vi "_readLabel_fromLabelList_wmg.vi"(0 "input_str_SN":string="8SSC10G59338L1DG5AN0004", 1 "input_str_PN":string="L01HE006-SD-R") -> (2 "show_str_SN":string, 3 "show_int_SN":i32, 4 "show_string_yydddXXXX":string, 5 "show_date":timestamp format="%<%X\n%x>T")   [LabVIEW 2011]
panel:
  in  "midVar_date_2":timestamp
  in  "midVar_date_1":timestamp
  # "周日是一周的第0天"
  # "1904050897/Z00A2R1543S500016\n0       5       10         17     22\nL99SF014-SD-H"
  # "8SSC10G59338L1DG5AN0004\nL01HE006-SD-R"
  # "1904050897/Z00A2R1543S500016\n0       5       10         17     22\nL99SF014-SD-H\n\n1543S5经本程序计算得到2015/10/23 296"
  # "8SSC10G59338L1DG5AN0004\n\nL01HE006-SD-R\n5AN经本程序计算得到2015/10/22 295\n\n8SSC10G59338L1DG5110004\nL01HE006-SD-R\n5AN经本程序计算得到2015/1/1 1"
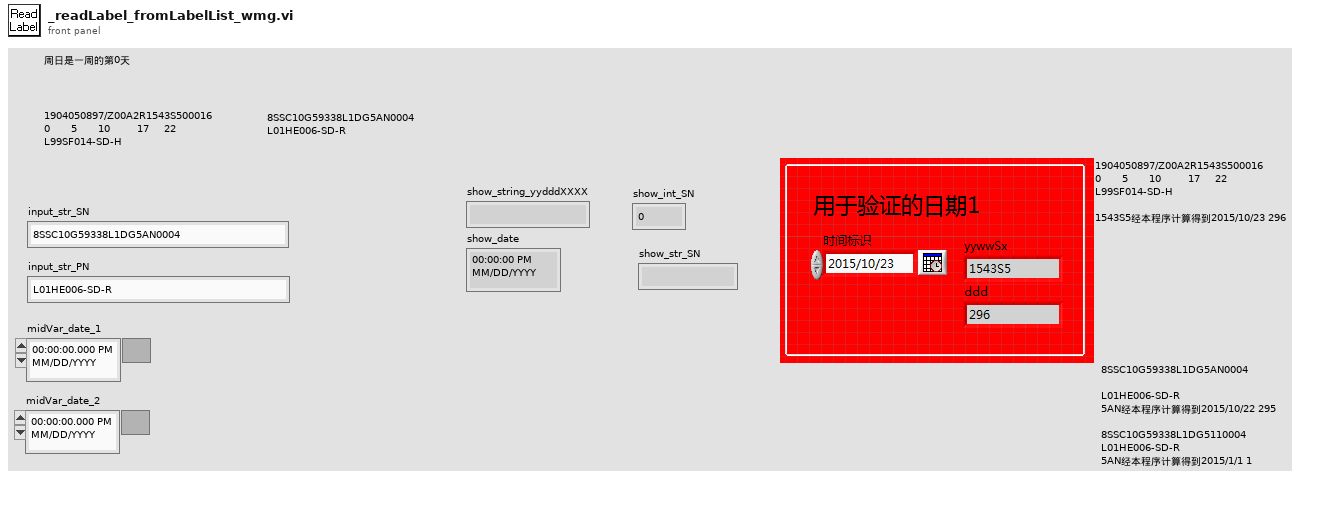
[diagram p1: front panel]
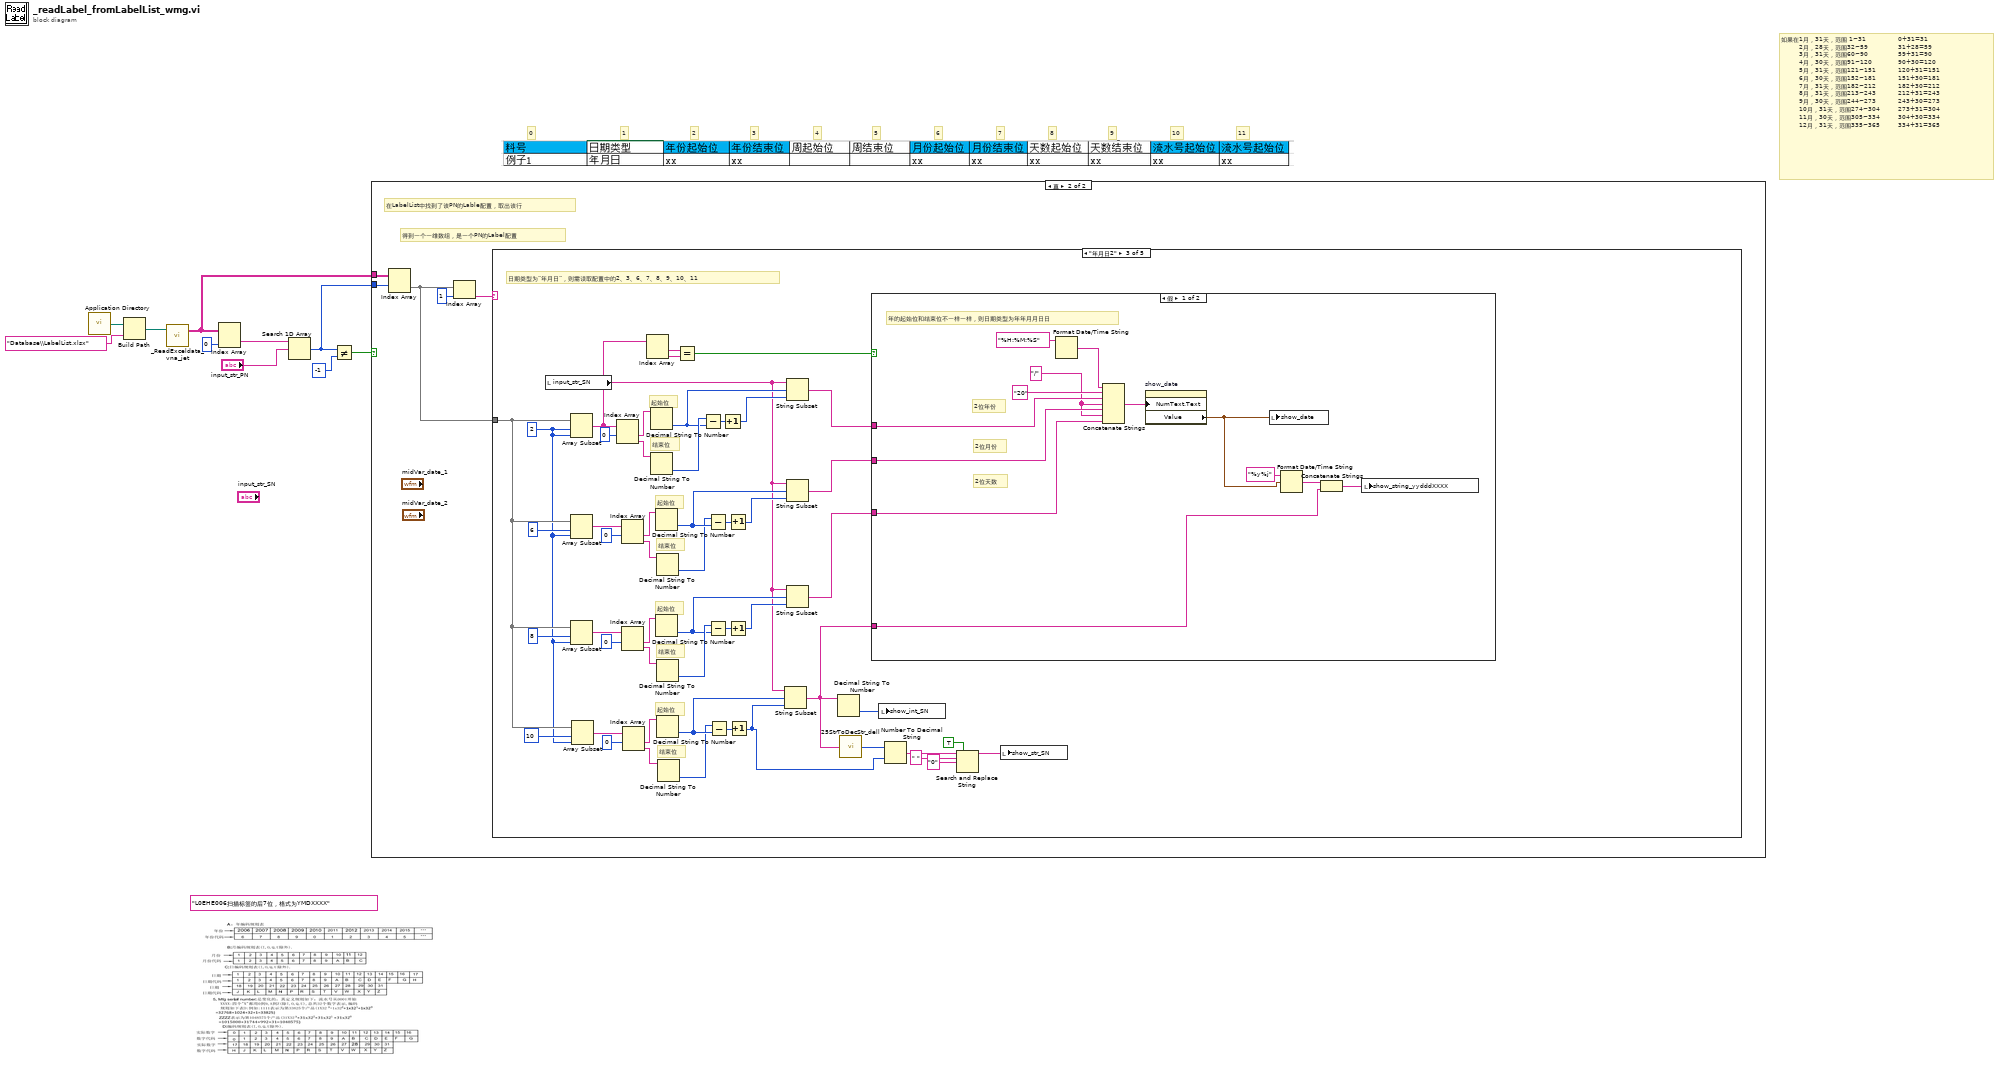
[diagram p0: block diagram]
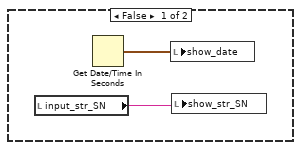
[diagram p2: hidden frame]
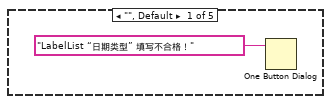
[diagram p3: hidden frame]
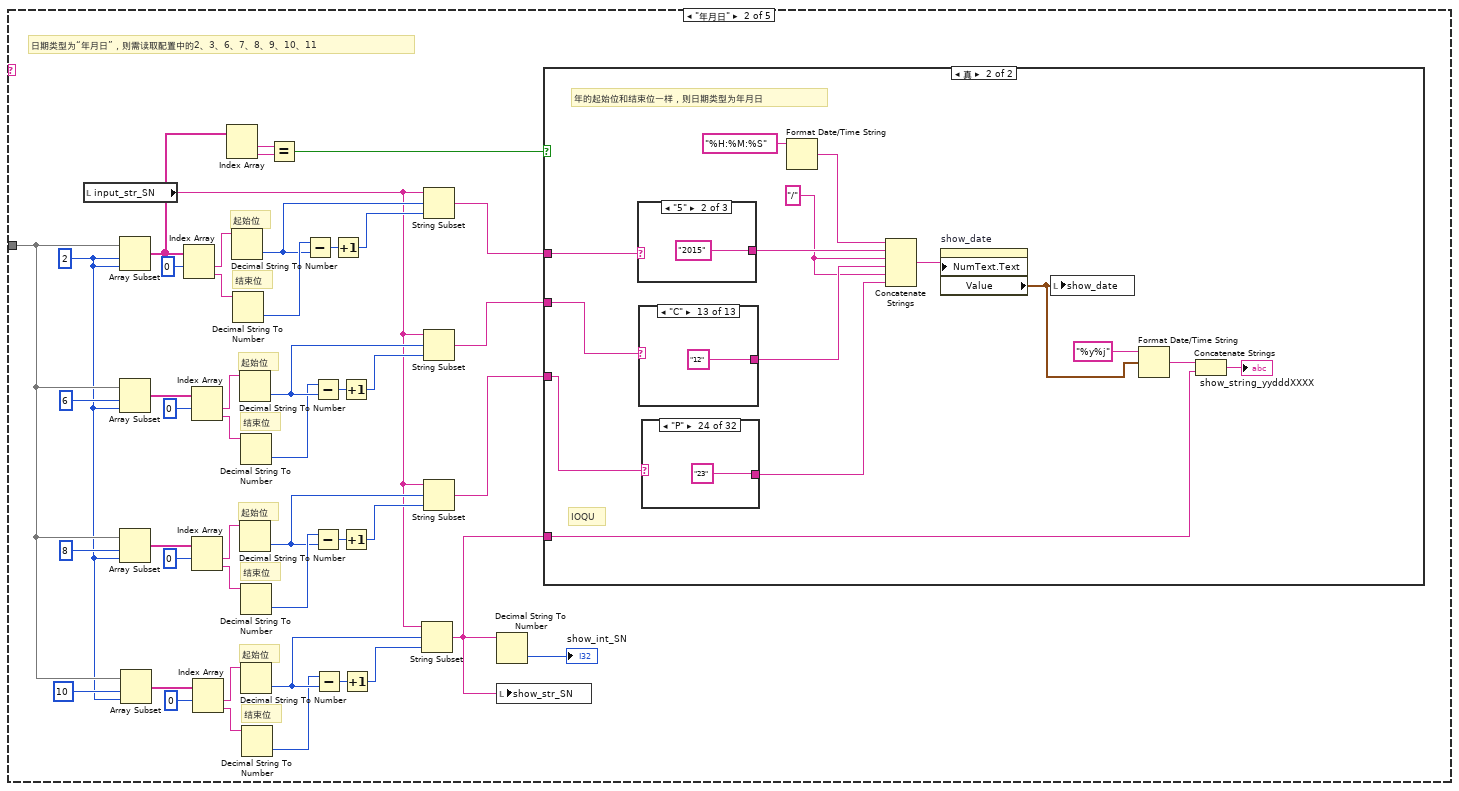
[diagram p4: hidden frame]
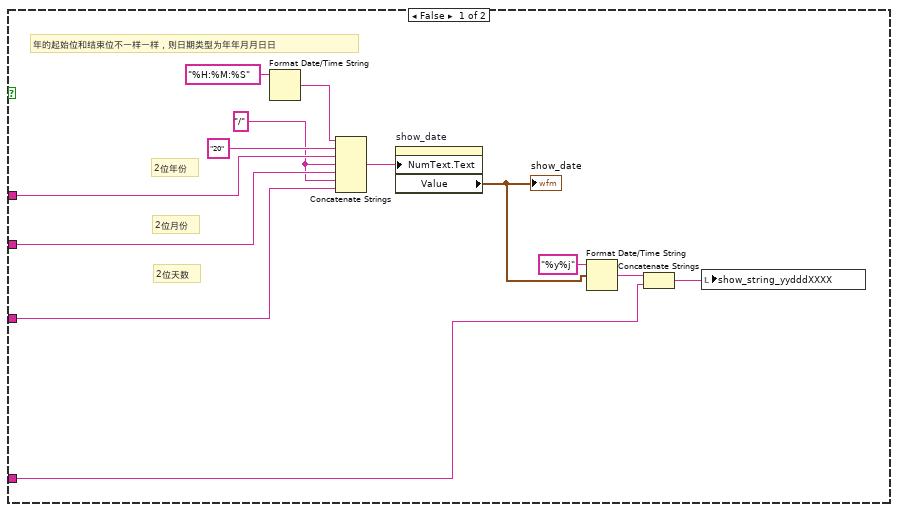
[diagram p5: hidden frame]
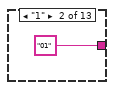
[diagram p7: hidden frame]
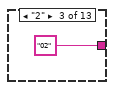
[diagram p8: hidden frame]
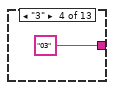
[diagram p9: hidden frame]
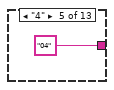
[diagram p10: hidden frame]
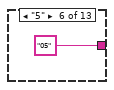
[diagram p11: hidden frame]
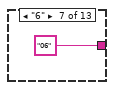
[diagram p12: hidden frame]
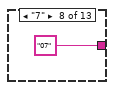
[diagram p13: hidden frame]
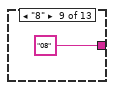
[diagram p14: hidden frame]
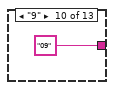
[diagram p15: hidden frame]
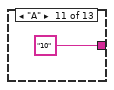
[diagram p16: hidden frame]
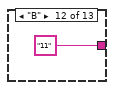
[diagram p17: hidden frame]
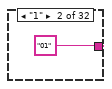
[diagram p19: hidden frame]
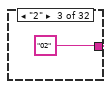
[diagram p20: hidden frame]
diagram:
  (unwired) "L0EHE006扫描标签的后7位，格式为YMDXXXX"
  # "如果在1月，31天，范围 1~31                0+31=31\n         2月，28天，范围32~59               31+28=59\n         3月，31天，范围60~90               59+31=90\n         4月，30天，范围91~120             90+30=120\n         5月，31天，范围121~151           120+31=151\n         6月，30天，范围152~181           151+30=181\n         7月，31天，范围182~212           182+30=212\n         8月，31天，范围213~243           212+31=243\n         9月，30天，范围244~273           243+30=273\n         10月，31天，范围274~304         273+31=304\n         11月，30天，范围305~334         304+30=334\n         12月，31天，范围335~365         334+31=365"
  # "11"
  # "10"
  # "9"
  # "8"
  # "7"
  # "6"
  # "5"
  # "4"
  # "3"
  # "2"
  # "1"
  # "0"
  n1 = call <vilib>:"Application Directory.vi"() -> ("Application Directory"=w10:path)
  n2 = Build Path(base path=w10, name or relative path="Database\\LabelList.xlsx") -> (appended path=w8:path)
  n3 = call "_ReadExceldata_vna_jet.vi"("路径"=w8) -> ("数据"=w2:string[][])  [unwired: 4 in]
  n4 = Index Array(array=w2, index (col)=0 ("禁用的索引 (列)")) -> (element=w6:string[])  [unwired: 1 in]
  n5 = Search 1D Array(1D array=w6, element="input_str_PN") -> (index of element=w1:i32)  [unwired: 1 in]
  n6 = Not Equal?(x=w1, y=-1) -> (x != y?=w3:bool)
  n7 = case shown="真" w3 {
    tunnel: w2 -> [_ w17]
    tunnel: w1 -> [_ w16]
    frame False {
      n8 = local read "input_str_SN"() -> (w11:string)
      n9 = Get Date/Time In Seconds() -> (seconds since 1Jan1904=w12:timestamp)
      n10 = local write "show_date"(w12) -> ()
      n11 = local write "show_str_SN"(w11) -> ()
    }
    frame True {
      # "得到一个一维数组，是一个PN的Label配置"
      # "在LabelList中找到了该PN的Lable配置，取出该行"
      n12 = Index Array(array=w17, index (row)=w16) -> (element=w13:string[])  [unwired: 1 in]
      n13 = Index Array(array=w13, index=1 ("索引")) -> (element=w14:string)
      n14 = case shown="\"年月日2\"" w14 {
        tunnel: w13 -> [_ w61 w186 w333 w357]
        frame "", Default {
          n15 = One Button Dialog(message="LabelList “日期类型” 填写不合格！") -> ()  [unwired: 1 in, 1 out]
        }
        frame "年月日" {
          w60 = 2 ("索引")
          # "结束位"
          # "起始位"
          # "结束位"
          # "起始位"
          # "结束位"
          # "起始位"
          # "结束位"
          # "起始位"
          # "日期类型为“年月日”，则需读取配置中的2、3、6、7、8、9、10、11"
          n16 = local read "input_str_SN"() -> (w21:string)
          n17 = Array Subset(array=w61, index=w60, length=w60) -> (w55:string[])
          n18 = Array Subset(array=w61, index=6 ("索引"), length=w60) -> (w42:string[])
          n19 = Array Subset(array=w61, index=8 ("索引"), length=w60) -> (w34:string[])
          n20 = Array Subset(array=w61, index=10 ("索引"), length=w60) -> (w22:string[])
          n21 = Index Array(array=w55, index #1=0 ("索引")) -> (element #1=w54:string, element #2=w53:string)  [unwired: 1 in]
          n22 = Index Array(array=w42, index #1=0 ("索引")) -> (element #1=w44:string, element #2=w45:string)  [unwired: 1 in]
          n23 = Index Array(array=w34, index #1=0 ("索引")) -> (element #1=w35:string, element #2=w39:string)  [unwired: 1 in]
          n24 = Index Array(array=w22, index #1=0 ("索引")) -> (element #1=w28:string, element #2=w24:string)  [unwired: 1 in]
          n25 = Index Array(array=w55) -> (element #1=w59:string, element #2=w58:string)  [unwired: 2 in]
          n26 = Decimal String To Number(string=w54) -> (number=w51:i32)  [unwired: 2 in, 1 out]
          n27 = Decimal String To Number(string=w53) -> (number=w52:i32)  [unwired: 2 in, 1 out]
          n28 = Decimal String To Number(string=w44) -> (number=w47:i32)  [unwired: 2 in, 1 out]
          n29 = Decimal String To Number(string=w35) -> (number=w37:i32)  [unwired: 2 in, 1 out]
          n30 = Decimal String To Number(string=w45) -> (number=w46:i32)  [unwired: 2 in, 1 out]
          n31 = Decimal String To Number(string=w39) -> (number=w38:i32)  [unwired: 2 in, 1 out]
          n32 = Decimal String To Number(string=w28) -> (number=w26:i32)  [unwired: 2 in, 1 out]
          n33 = Decimal String To Number(string=w24) -> (number=w25:i32)  [unwired: 2 in, 1 out]
          n34 = Equal?(x=w59, y=w58) -> (x = y?=w57:bool)
          n35 = Subtract(x=w52, y=w51) -> (x-y=w56:i32)
          n36 = Subtract(x=w46, y=w47) -> (x-y=w43:i32)
          n37 = Subtract(x=w38, y=w37) -> (x-y=w40:i32)
          n38 = Subtract(x=w25, y=w26) -> (x-y=w23:i32)
          n39 = Increment(x=w56) -> (x+1=w50:i32)
          n40 = Increment(x=w43) -> (x+1=w48:i32)
          n41 = Increment(x=w40) -> (x+1=w36:i32)
          n42 = Increment(x=w23) -> (x+1=w27:i32)
          n43 = String Subset(string=w21, offset (0)=w26, length (rest)=w27) -> (substring=w19:string)
          n44 = String Subset(string=w21, offset (0)=w51, length (rest)=w50) -> (substring=w49:string)
          n45 = String Subset(string=w21, offset (0)=w47, length (rest)=w48) -> (substring=w41:string)
          n46 = String Subset(string=w21, offset (0)=w37, length (rest)=w36) -> (substring=w30:string)
          n47 = Decimal String To Number(string=w19) -> (number=→"show_int_SN":i32)  [unwired: 2 in, 1 out]
          n48 = local write "show_str_SN"(w19) -> ()
          n49 = case shown="真" w57 {
            tunnel: w49 -> [w76 w92]
            tunnel: w41 -> [w75 w90]
            tunnel: w30 -> [w73 w91]
            tunnel: w19 -> [w65 w78]
            frame False {
              w74 = "/"
              # "年的起始位和结束位不一样一样，则日期类型为年年月月日日"
              # "2位天数"
              # "2位月份"
              # "2位年份"
              n50 = Format Date/Time String(time format string (%c)="%H:%M:%S" ("时间格式字符串(%c)")) -> (date/time string=w71:string)  [unwired: 2 in]
              n51 = Concatenate Strings(w71, "20", w76, w74, w75, w74, w73) -> (w70:string)
              n52 = property on="show_date" class="AbsTime (严格)"("NumText.Text"=w70) -> ("Value"=w66:timestamp)  [unwired: 2 in, 2 out]
              "show_date" <- w66
              n53 = Format Date/Time String(time format string (%c)="%y%j" ("时间格式字符串(%c)"), seconds (now)=w66) -> (date/time string=w68:string)  [unwired: 1 in]
              n54 = Concatenate Strings(w68, w65) -> (w69:string)
              n55 = local write "show_string_yydddXXXX"(w69) -> ()
            }
            frame True {
              w85 = "/"
              # "IOQU"
              # "年的起始位和结束位一样，则日期类型为年月日"
              n56 = case shown="\"5\"" w92 {
                tunnel: [_ "2015" "2016"] -> w89
                frame Default {
                }
                frame "5" {
                }
                frame "6" {
                }
              }
              n57 = case shown="\"C\"" w90 {
                tunnel: [_ "01" "02" "03" "04" "05" "06" "07" "08" "09" "10" "11" "12"] -> w86
                frame "", Default {
                }
                frame "1" {
                }
                frame "2" {
                }
                frame "3" {
                }
                frame "4" {
                }
                frame "5" {
                }
                frame "6" {
                }
                frame "7" {
                }
                frame "8" {
                }
                frame "9" {
                }
                frame "A" {
                }
                frame "B" {
                }
                frame "C" {
                }
              }
              n58 = case shown="\"P\"" w91 {
                tunnel: [_ "01" "02" "03" "04" "05" "06" "07" "08" "09" "10" "11" "12" "13" "14" "15" "16" "17" "18" "19" "20" "21" "22" "23" "24" "25" "26" "27" "28" "29" "30" "31"] -> w84
                frame "", Default {
                }
                frame "1" {
                }
                frame "2" {
                }
                frame "3" {
                }
                frame "4" {
                }
                frame "5" {
                }
                frame "6" {
                }
                frame "7" {
                }
                frame "8" {
                }
                frame "9" {
                }
                frame "A" {
                }
                frame "B" {
                }
                frame "C" {
                }
                frame "D" {
                }
                frame "E" {
                }
                frame "F" {
                }
                frame "G" {
                }
                frame "H" {
                }
                frame "J" {
                }
                frame "K" {
                }
                frame "L" {
                }
                frame "M" {
                }
                frame "N" {
                }
                frame "P" {
                }
                frame "R" {
                }
                frame "S" {
                }
                frame "T" {
                }
                frame "V" {
                }
                frame "W" {
                }
                frame "X" {
                }
                frame "Y" {
                }
                frame "Z" {
                }
              }
              n59 = Format Date/Time String(time format string (%c)="%H:%M:%S" ("时间格式字符串(%c)")) -> (date/time string=w87:string)  [unwired: 2 in]
              n60 = Concatenate Strings(w87, w89, w85, w86, w85, w84) -> (w83:string)
              n61 = property on="show_date" class="AbsTime (严格)"("NumText.Text"=w83) -> ("Value"=w79:timestamp)  [unwired: 2 in, 2 out]
              n62 = local write "show_date"(w79) -> ()
              n63 = Format Date/Time String(time format string (%c)="%y%j" ("时间格式字符串(%c)"), seconds (now)=w79) -> (date/time string=w81:string)  [unwired: 1 in]
              n64 = Concatenate Strings(w81, w78) -> (→"show_string_yydddXXXX":string)
            }
          }
        }
        frame "年月日2" {
          w185 = 2 ("索引")
          # "结束位"
          # "起始位"
          # "结束位"
          # "起始位"
          # "结束位"
          # "起始位"
          # "结束位"
          # "起始位"
          # "日期类型为“年月日”，则需读取配置中的2、3、6、7、8、9、10、11"
          n65 = local read "input_str_SN"() -> (w147:string)
          n66 = Array Subset(array=w186, index=w185, length=w185) -> (w180:string[])
          n67 = Array Subset(array=w186, index=6 ("索引"), length=w185) -> (w167:string[])
          n68 = Array Subset(array=w186, index=8 ("索引"), length=w185) -> (w159:string[])
          n69 = Array Subset(array=w186, index=10 ("索引"), length=w185) -> (w148:string[])
          n70 = Index Array(array=w180, index #1=0 ("索引")) -> (element #1=w179:string, element #2=w178:string)  [unwired: 1 in]
          n71 = Index Array(array=w167, index #1=0 ("索引")) -> (element #1=w169:string, element #2=w170:string)  [unwired: 1 in]
          n72 = Index Array(array=w159, index #1=0 ("索引")) -> (element #1=w160:string, element #2=w164:string)  [unwired: 1 in]
          n73 = Index Array(array=w148, index #1=0 ("索引")) -> (element #1=w153:string, element #2=w150:string)  [unwired: 1 in]
          n74 = Index Array(array=w180) -> (element #1=w184:string, element #2=w183:string)  [unwired: 2 in]
          n75 = Decimal String To Number(string=w179) -> (number=w176:i32)  [unwired: 2 in, 1 out]
          n76 = Decimal String To Number(string=w178) -> (number=w177:i32)  [unwired: 2 in, 1 out]
          n77 = Decimal String To Number(string=w169) -> (number=w172:i32)  [unwired: 2 in, 1 out]
          n78 = Decimal String To Number(string=w160) -> (number=w162:i32)  [unwired: 2 in, 1 out]
          n79 = Decimal String To Number(string=w170) -> (number=w171:i32)  [unwired: 2 in, 1 out]
          n80 = Decimal String To Number(string=w164) -> (number=w163:i32)  [unwired: 2 in, 1 out]
          n81 = Decimal String To Number(string=w153) -> (number=w152:i32)  [unwired: 2 in, 1 out]
          n82 = Decimal String To Number(string=w150) -> (number=w151:i32)  [unwired: 2 in, 1 out]
          n83 = Equal?(x=w184, y=w183) -> (x = y?=w182:bool)
          n84 = Subtract(x=w177, y=w176) -> (x-y=w181:i32)
          n85 = Subtract(x=w171, y=w172) -> (x-y=w168:i32)
          n86 = Subtract(x=w163, y=w162) -> (x-y=w165:i32)
          n87 = Subtract(x=w151, y=w152) -> (x-y=w149:i32)
          n88 = Increment(x=w181) -> (x+1=w175:i32)
          n89 = Increment(x=w168) -> (x+1=w173:i32)
          n90 = Increment(x=w165) -> (x+1=w161:i32)
          n91 = Increment(x=w149) -> (x+1=w143:i32)
          n92 = String Subset(string=w147, offset (0)=w152, length (rest)=w143) -> (substring=w146:string)
          n93 = String Subset(string=w147, offset (0)=w176, length (rest)=w175) -> (substring=w174:string)
          n94 = String Subset(string=w147, offset (0)=w172, length (rest)=w173) -> (substring=w166:string)
          n95 = String Subset(string=w147, offset (0)=w162, length (rest)=w161) -> (substring=w155:string)
          n96 = Decimal String To Number(string=w146) -> (number=w145:i32)  [unwired: 2 in, 1 out]
          n97 = call "25StrToDecStr_dell.vi"("input_str_hex"=w146) -> ("数值"=w144:i32)
          n98 = case shown="假" w182 {
            tunnel: w174 -> [w201 w217]
            tunnel: w166 -> [w200 w215]
            tunnel: w155 -> [w198 w216]
            tunnel: w146 -> [w192 w204]
            frame False {
              w199 = "/"
              # "年的起始位和结束位不一样一样，则日期类型为年年月月日日"
              # "2位天数"
              # "2位月份"
              # "2位年份"
              n99 = Format Date/Time String(time format string (%c)="%H:%M:%S" ("时间格式字符串(%c)")) -> (date/time string=w196:string)  [unwired: 2 in]
              n100 = Concatenate Strings(w196, "20", w201, w199, w200, w199, w198) -> (w195:string)
              n101 = property on="show_date" class="AbsTime (严格)"("NumText.Text"=w195) -> ("Value"=w191:timestamp)  [unwired: 2 in, 2 out]
              n102 = local write "show_date"(w191) -> ()
              n103 = Format Date/Time String(time format string (%c)="%y%j" ("时间格式字符串(%c)"), seconds (now)=w191) -> (date/time string=w194:string)  [unwired: 1 in]
              n104 = Concatenate Strings(w194, w192) -> (w190:string)
              n105 = local write "show_string_yydddXXXX"(w190) -> ()
            }
            frame True {
              w210 = "/"
              # "WXYZ"
              # "年的起始位和结束位一样，则日期类型为年月日"
              n106 = case shown="\"5\"" w217 {
                tunnel: [_ "2015" "2016"] -> w214
                frame Default {
                }
                frame "5" {
                }
                frame "6" {
                }
              }
              n107 = case shown="\"C\"" w215 {
                tunnel: [_ "01" "02" "03" "04" "05" "06" "07" "08" "09" "10" "11" "12"] -> w211
                frame "", Default {
                }
                frame "1" {
                }
                frame "2" {
                }
                frame "3" {
                }
                frame "4" {
                }
                frame "5" {
                }
                frame "6" {
                }
                frame "7" {
                }
                frame "8" {
                }
                frame "9" {
                }
                frame "A" {
                }
                frame "B" {
                }
                frame "C" {
                }
              }
              n108 = case shown="\"R\"" w216 {
                tunnel: [_ "01" "02" "03" "04" "05" "06" "07" "08" "09" "10" "11" "12" "13" "14" "15" "16" "17" "18" "19" "20" "21" "22" "23" "24" "25" "26" "27" "28" "29" "30" "31"] -> w209
                frame "", Default {
                }
                frame "1" {
                }
                frame "2" {
                }
                frame "3" {
                }
                frame "4" {
                }
                frame "5" {
                }
                frame "6" {
                }
                frame "7" {
                }
                frame "8" {
                }
                frame "9" {
                }
                frame "A" {
                }
                frame "B" {
                }
                frame "C" {
                }
                frame "D" {
                }
                frame "E" {
                }
                frame "F" {
                }
                frame "G" {
                }
                frame "H" {
                }
                frame "I" {
                }
                frame "J" {
                }
                frame "K" {
                }
                frame "L" {
                }
                frame "M" {
                }
                frame "N" {
                }
                frame "O" {
                }
                frame "P" {
                }
                frame "Q" {
                }
                frame "R" {
                }
                frame "S" {
                }
                frame "T" {
                }
                frame "U" {
                }
                frame "V" {
                }
              }
              n109 = Format Date/Time String(time format string (%c)="%H:%M:%S" ("时间格式字符串(%c)")) -> (date/time string=w212:string)  [unwired: 2 in]
              n110 = Concatenate Strings(w212, w214, w210, w211, w210, w209) -> (w208:string)
              n111 = property on="show_date" class="AbsTime (严格)"("NumText.Text"=w208) -> ("Value"=w205:timestamp)  [unwired: 2 in, 2 out]
              n112 = local write "show_date"(w205) -> ()
              n113 = Format Date/Time String(time format string (%c)="%y%j" ("时间格式字符串(%c)"), seconds (now)=w205) -> (date/time string=w206:string)  [unwired: 1 in]
              n114 = Concatenate Strings(w206, w204) -> (w203:string)
              n115 = local write "show_string_yydddXXXX"(w203) -> ()
            }
          }
          n116 = local write "show_int_SN"(w145) -> ()
          n117 = Number To Decimal String(number=w144, width (-)=w143) -> (decimal integer string=w142:string)
          n118 = Search and Replace String(replace all?=TRUE ("替换全部？(F)"), input string=w142, search string=" " ("搜索字符串"), replace string="0" ("替换字符串(\"\")")) -> (result string=w138:string)  [unwired: 4 in, 3 out]
          n119 = local write "show_str_SN"(w138) -> ()
        }
        frame "年周" {
          w305 = "/"
          w332 = 2 ("索引")
          # "得到本周一在本月的天数"
          # "减去首尾周的天数"
          # "如何由周数+本周一计算出本月天数？\n由周数-2，加本周周一，计算出天数，\n然后减去上个月的天数"
          # "如何由周数计算出月份？\n由周数-2，加本周周一，计算出天数\n再根据12月份的天数范围去匹配"
          # "日期类型为“年周”实际是“年年周周”，天数按照当天去补"
          # "2位天数"
          # "2位周数"
          # "2位年份"
          # "日期类型为“年周”，则需读取配置中的2、3、4、5、10、11"
          # "结束位"
          # "起始位"
          # "结束位"
          # "起始位"
          # "结束位"
          # "起始位"
          n120 = local read "input_str_SN"() -> (w307:string)
          n121 = Array Subset(array=w333, index=w332, length=w332) -> (w301:string[])
          n122 = Array Subset(array=w333, index=4 ("索引"), length=w332) -> (w318:string[])
          n123 = Array Subset(array=w333, index=10 ("索引"), length=w332) -> (w308:string[])
          n124 = Index Array(array=w301, index #1=0 ("索引")) -> (element #1=w330:string, element #2=w329:string)  [unwired: 1 in]
          n125 = Index Array(array=w318, index #1=0 ("索引")) -> (element #1=w320:string, element #2=w321:string)  [unwired: 1 in]
          n126 = Index Array(array=w308, index #1=0 ("索引")) -> (element #1=w314:string, element #2=w310:string)  [unwired: 1 in]
          n127 = Decimal String To Number(string=w330) -> (number=w327:i32)  [unwired: 2 in, 1 out]
          n128 = Decimal String To Number(string=w329) -> (number=w328:i32)  [unwired: 2 in, 1 out]
          n129 = Decimal String To Number(string=w320) -> (number=w323:i32)  [unwired: 2 in, 1 out]
          n130 = Decimal String To Number(string=w321) -> (number=w322:i32)  [unwired: 2 in, 1 out]
          n131 = Decimal String To Number(string=w314) -> (number=w312:i32)  [unwired: 2 in, 1 out]
          n132 = Decimal String To Number(string=w310) -> (number=w311:i32)  [unwired: 2 in, 1 out]
          n133 = Subtract(x=w328, y=w327) -> (x-y=w331:i32)
          n134 = Subtract(x=w322, y=w323) -> (x-y=w319:i32)
          n135 = Subtract(x=w311, y=w312) -> (x-y=w309:i32)
          n136 = Increment(x=w331) -> (x+1=w326:i32)
          n137 = Increment(x=w319) -> (x+1=w324:i32)
          n138 = Increment(x=w309) -> (x+1=w313:i32)
          n139 = String Subset(string=w307, offset (0)=w312, length (rest)=w313) -> (substring=w263:string)
          "show_str_SN" <- w263
          n140 = String Subset(string=w307, offset (0)=w327, length (rest)=w326) -> (substring=w325:string)
          n141 = String Subset(string=w307, offset (0)=w323, length (rest)=w324) -> (substring=w299:string)
          n142 = Decimal String To Number(string=w263) -> (number=w267:i32)  [unwired: 2 in, 1 out]
          n143 = Decimal String To Number(string=w299) -> (number=w288:i32)  [unwired: 2 in, 1 out]
          n144 = Format Date/Time String(time format string (%c)="20:15:00\n%Y/01/01" ("时间格式字符串(%c)")) -> (date/time string=w295:string)  [unwired: 2 in]
          n145 = local write "show_int_SN"(w267) -> ()
          n146 = Subtract(x=w288, y=2) -> (x-y=w298:i32)
          n147 = property on="midVar_date_1" class="AbsTime (严格)"("NumText.Text"=w295) -> ("Value"=w294:timestamp)  [unwired: 2 in, 2 out]
          n148 = Multiply(x=w298, y=7) -> (x*y=w286:i32)
          n149 = Format Date/Time String(time format string (%c)="%w" ("时间格式字符串(%c)"), seconds (now)=w294) -> (date/time string=w291:string)  [unwired: 1 in]
          n150 = Decimal String To Number(string=w291) -> (number=w290:i32)  [unwired: 2 in, 1 out]
          n151 = Subtract(x=7, y=w290) -> (x-y=w289:i32)
          n152 = Increment(x=w289) -> (x+1=w285:i32)
          n153 = Compound Arithmetic op=ADD(w286, w285, 1 ("值")) -> (w275:i32)
          n154 = Format Date/Time String(time format string (%c)="%Y/" ("时间格式字符串(%c)")) -> (date/time string=w282:string)  [unwired: 2 in]
          n155 = case shown="335..365" w275 {
            tunnel: ["01" "02" "03" "04" "05" "06" "07" "08" "09" "10" "11" "12"] -> w265
            frame 1..31, Default {
            }
            frame 32..59 {
            }
            frame 60..90 {
            }
            frame 91..120 {
            }
            frame 121..151 {
            }
            frame 152..181 {
            }
            frame 182..212 {
            }
            frame 213..243 {
            }
            frame 244..273 {
            }
            frame 274..304 {
            }
            frame 305..334 {
            }
            frame 335..365 {
            }
          }
          n156 = Format Date/Time String(time format string (%c)="%H:%M:%S" ("时间格式字符串(%c)")) -> (date/time string=w279:string)  [unwired: 2 in]
          n157 = Concatenate Strings(w279, w282, w265, "/01") -> (w280:string)
          n158 = property on="midVar_date_2" class="AbsTime (严格)"("NumText.Text"=w280) -> ("Value"=w278:timestamp)  [unwired: 2 in, 2 out]
          n159 = Format Date/Time String(time format string (%c)="%j" ("时间格式字符串(%c)"), seconds (now)=w278) -> (date/time string=w276:string)  [unwired: 1 in]
          n160 = Decimal String To Number(string=w276) -> (number=w274:i32)  [unwired: 2 in, 1 out]
          n161 = Decrement(x=w274) -> (x-1=w264:i32)
          n162 = Format Date/Time String(time format string (%c)="%H:%M:%S" ("时间格式字符串(%c)")) -> (date/time string=w303:string)  [unwired: 2 in]
          n163 = Subtract(x=w275, y=w264) -> (x-y=w273:i32)
          n164 = call "intToNWidthString.vi"("input_int_width"=2, "input_int_number"=w273) -> ("show_str_number"=w272:string)
          n165 = Concatenate Strings(w303, "20", w325, w305, w265, w305, w272) -> (w302:string)
          n166 = property on="show_date" class="AbsTime (严格)"("NumText.Text"=w302) -> ("Value"=w268:timestamp)  [unwired: 2 in, 2 out]
          n167 = Format Date/Time String(time format string (%c)="%y%j" ("时间格式字符串(%c)"), seconds (now)=w268) -> (date/time string=w270:string)  [unwired: 1 in]
          n168 = Concatenate Strings(w270, w263) -> (w269:string)
          n169 = local write "show_date"(w268) -> ()
          n170 = local write "show_string_yydddXXXX"(w269) -> ()
        }
        frame "年周天" {
          w404 = "/"
          w356 = 2 ("索引")
          # "如何计算之前月份的所有天数？\n用本月1号来算，结果减去1即可"
          # "结束位"
          # "起始位"
          # "得到本周一在本月的天数"
          # "减去首尾周的天数"
          # "如何由周数+本周一计算出本月天数？\n由周数-2，加本周周一，计算出天数，\n然后减去前所有月的天数"
          # "如何由周数计算出月份？\n由周数-2，加本周周一，计算出天数\n再根据12月份的天数范围去匹配"
          # "日期类型为“年周天”实际是“年年周周天”"
          # "2位天数"
          # "2位周数"
          # "2位年份"
          # "日期类型为“年周天”，则需读取配置中的2、3、4、5、8、9、10、11"
          # "结束位"
          # "起始位"
          # "结束位"
          # "起始位"
          # "结束位"
          # "起始位"
          n171 = local read "input_str_SN"() -> (w355:string)
          n172 = Array Subset(array=w357, index=8 ("索引"), length=w356) -> (w365:string[])
          n173 = Array Subset(array=w357, index=w356, length=w356) -> (w401:string[])
          n174 = Array Subset(array=w357, index=4 ("索引"), length=w356) -> (w416:string[])
          n175 = Array Subset(array=w357, index=10 ("索引"), length=w356) -> (w406:string[])
          n176 = Index Array(array=w401, index #1=0 ("索引")) -> (element #1=w428:string, element #2=w427:string)  [unwired: 1 in]
          n177 = Index Array(array=w365, index #1=0 ("索引")) -> (element #1=w363:string, element #2=w362:string)  [unwired: 1 in]
          n178 = Index Array(array=w416, index #1=0 ("索引")) -> (element #1=w418:string, element #2=w419:string)  [unwired: 1 in]
          n179 = Index Array(array=w406, index #1=0 ("索引")) -> (element #1=w412:string, element #2=w408:string)  [unwired: 1 in]
          n180 = Decimal String To Number(string=w428) -> (number=w425:i32)  [unwired: 2 in, 1 out]
          n181 = Decimal String To Number(string=w427) -> (number=w426:i32)  [unwired: 2 in, 1 out]
          n182 = Decimal String To Number(string=w363) -> (number=w360:i32)  [unwired: 2 in, 1 out]
          n183 = Decimal String To Number(string=w418) -> (number=w421:i32)  [unwired: 2 in, 1 out]
          n184 = Decimal String To Number(string=w362) -> (number=w361:i32)  [unwired: 2 in, 1 out]
          n185 = Decimal String To Number(string=w419) -> (number=w420:i32)  [unwired: 2 in, 1 out]
          n186 = Decimal String To Number(string=w412) -> (number=w410:i32)  [unwired: 2 in, 1 out]
          n187 = Decimal String To Number(string=w408) -> (number=w409:i32)  [unwired: 2 in, 1 out]
          n188 = Subtract(x=w426, y=w425) -> (x-y=w429:i32)
          n189 = Subtract(x=w361, y=w360) -> (x-y=w364:i32)
          n190 = Subtract(x=w420, y=w421) -> (x-y=w417:i32)
          n191 = Subtract(x=w409, y=w410) -> (x-y=w407:i32)
          n192 = Increment(x=w429) -> (x+1=w424:i32)
          n193 = Increment(x=w364) -> (x+1=w359:i32)
          n194 = Increment(x=w417) -> (x+1=w422:i32)
          n195 = Increment(x=w407) -> (x+1=w411:i32)
          n196 = String Subset(string=w355, offset (0)=w410, length (rest)=w411) -> (substring=w348:string)
          n197 = String Subset(string=w355, offset (0)=w360, length (rest)=w359) -> (substring=w354:string)
          n198 = String Subset(string=w355, offset (0)=w425, length (rest)=w424) -> (substring=w423:string)
          n199 = String Subset(string=w355, offset (0)=w421, length (rest)=w422) -> (substring=w399:string)
          n200 = Decimal String To Number(string=w348) -> (number=w368:i32)  [unwired: 2 in, 1 out]
          n201 = Decimal String To Number(string=w399) -> (number=w388:i32)  [unwired: 2 in, 1 out]
          n202 = Decimal String To Number(string=w354) -> (number=w353:i32)  [unwired: 2 in, 1 out]
          n203 = Format Date/Time String(time format string (%c)="20:15:00\n%Y/01/01" ("时间格式字符串(%c)")) -> (date/time string=w395:string)  [unwired: 2 in]
          n204 = local write "show_int_SN"(w368) -> ()
          n205 = Subtract(x=w388, y=2) -> (x-y=w398:i32)
          n206 = property on="midVar_date_1" class="AbsTime (严格)"("NumText.Text"=w395) -> ("Value"=w394:timestamp)  [unwired: 2 in, 2 out]
          n207 = Multiply(x=w398, y=7) -> (x*y=w386:i32)
          n208 = Format Date/Time String(time format string (%c)="%w" ("时间格式字符串(%c)"), seconds (now)=w394) -> (date/time string=w391:string)  [unwired: 1 in]
          n209 = Decimal String To Number(string=w391) -> (number=w390:i32)  [unwired: 2 in, 1 out]
          n210 = Subtract(x=7, y=w390) -> (x-y=w389:i32)
          n211 = Increment(x=w389) -> (x+1=w385:i32)
          n212 = Compound Arithmetic op=ADD(w386, w385, w353) -> (w376:i32)
          n213 = Format Date/Time String(time format string (%c)="%Y/" ("时间格式字符串(%c)")) -> (date/time string=w383:string)  [unwired: 2 in]
          n214 = case shown="335..365" w376 {
            tunnel: ["01" "02" "03" "04" "05" "06" "07" "08" "09" "10" "11" "12"] -> w352
            frame 1..31, Default {
            }
            frame 32..59 {
            }
            frame 60..90 {
            }
            frame 91..120 {
            }
            frame 121..151 {
            }
            frame 152..181 {
            }
            frame 182..212 {
            }
            frame 213..243 {
            }
            frame 244..273 {
            }
            frame 274..304 {
            }
            frame 305..334 {
            }
            frame 335..365 {
            }
          }
          n215 = Format Date/Time String(time format string (%c)="%H:%M:%S" ("时间格式字符串(%c)")) -> (date/time string=w380:string)  [unwired: 2 in]
          n216 = Concatenate Strings(w380, w383, w352, "/01") -> (w381:string)
          n217 = property on="midVar_date_2" class="AbsTime (严格)"("NumText.Text"=w381) -> ("Value"=w379:timestamp)  [unwired: 2 in, 2 out]
          n218 = Format Date/Time String(time format string (%c)="%j" ("时间格式字符串(%c)"), seconds (now)=w379) -> (date/time string=w377:string)  [unwired: 1 in]
          n219 = Decimal String To Number(string=w377) -> (number=w375:i32)  [unwired: 2 in, 1 out]
          n220 = Format Date/Time String(time format string (%c)="%H:%M:%S" ("时间格式字符串(%c)")) -> (date/time string=w350:string)  [unwired: 2 in]
          n221 = Decrement(x=w375) -> (x-1=w351:i32)
          n222 = Subtract(x=w376, y=w351) -> (x-y=w374:i32)
          n223 = call "intToNWidthString.vi"("input_int_width"=2, "input_int_number"=w374) -> ("show_str_number"=w373:string)
          n224 = Concatenate Strings(w350, "\n", "20", w423, w404, w352, w404, w373) -> (w402:string)
          n225 = property on="show_date" class="AbsTime (严格)"("NumText.Text"=w402) -> ("Value"=w369:timestamp)  [unwired: 2 in, 2 out]
          n226 = Format Date/Time String(time format string (%c)="%y%j" ("时间格式字符串(%c)"), seconds (now)=w369) -> (date/time string=w371:string)  [unwired: 1 in]
          n227 = Concatenate Strings(w371, w348) -> (w370:string)
          n228 = local write "show_str_SN"(w348) -> ()
          n229 = local write "show_string_yydddXXXX"(w370) -> ()
          n230 = local write "show_date"(w369) -> ()
        }
      }
    }
  }
